vi "Store Measurement.vi"(8 "error in (no error)":errorcluster, 9 "Value":string, 10 "Measurement Name":string, 11 "SCADA in":refnum<class "SCADA.lvclass">) -> (0 "error out":errorcluster, 3 "SCADA out":refnum<class "SCADA.lvclass">)   [LabVIEW 2015, in "SCADA Core.lvlib" / "SCADA.lvclass"]
uses:
  SCADA.lvclass
  SCADA.lvclass/SCADA.ctl
  <vilib>/NI/Tools/Keyed Array/Map String.vi
  <vilib>/NI/Tools/String/Get Case Matching.vi
  <vilib>/NI/Tools/Keyed Array/Tools_KeyedArray.lvlib
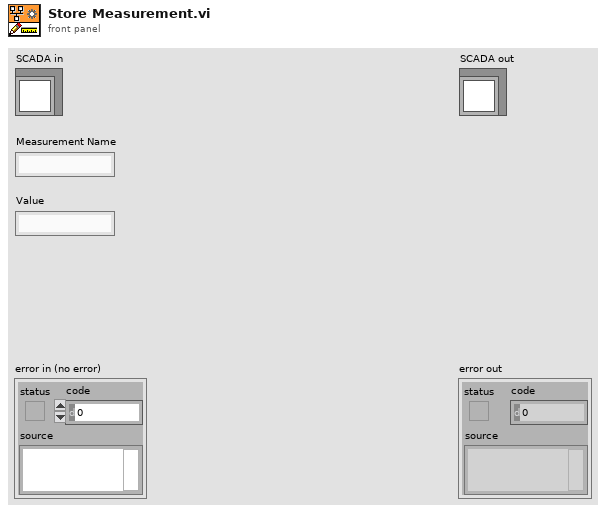
[diagram p1: front panel]
types:
  T1 = typedef "Tools_KeyedArray.lvlib/KeyedArray.ctl" = cluster{"keys":string[], "values":string[]}
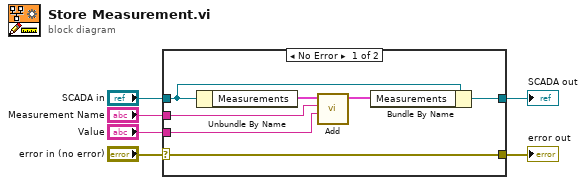
[diagram p0: block diagram]
diagram:
  n1 = case shown="No Error" "error in (no error)" {
    selector: "error in (no error)" -> [w13 w15]
    tunnel: [w13 w15] -> w5
    tunnel: [w9 w14] -> w3
    tunnel: "SCADA in" -> [w12 w14]
    tunnel: "Measurement Name" -> [w11 _]
    tunnel: "Value" -> [w10 _]
    frame No Error {
      n2 = Unbundle By Name(w12) -> ("Measurements"=w8:T1)
      n3 = call <vilib>:"Add.vi"("value"=w10, "key"=w11, "array in"=w8) -> ("array out"=w7:T1)  [unwired: 2 in, 2 out]
      n4 = Bundle By Name(cluster=w12, "Measurements"=w7) -> (w9:refnum<class "SCADA.lvclass">)
    }
    frame Error {
    }
  }
  "error out" <- w5
  "SCADA out" <- w3
